vi "Узел обратной связи.vi"() -> ()   [LabVIEW 2017]
doc: "This VI is an exercise in the LabVIEW Basics I course.\n\nIt is used to demonstrate the use of shift registers and feedback nodes. This VI initiallizes a Feedback Node with 1 then multiplies the feedback by 2. Open the block diagram to understand the two methods used."
panel:
  out "Feedback до":dbl
  out "Feedback после":dbl
  # "Этот ВП демонстрирует два способа использования узла обратной связи (Feedback Node). \n \nВ первом случае узел обратной связи отрабатывается после элемента отображения значений функции.\n\nВо втором случае узел обратной связи отрабатывается до элемента отображения значений функции."
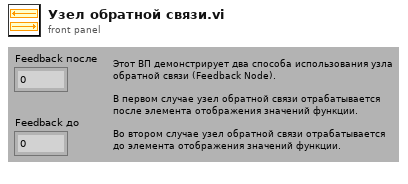
[diagram p1: front panel]
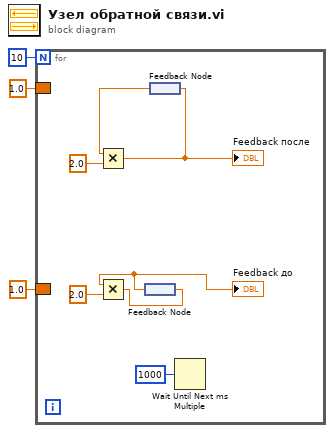
[diagram p0: block diagram]
diagram:
  n1 = for {
    N: 10 -> [_]
    border: 1.0 -> [_]
    border: 1.0 -> [_]
    n2 = feedback #1() -> (w5:dbl)
    "Feedback до" <- w5
    n3 = Multiply(x=w5, y=2.0) -> (x*y=w7:dbl)
    n4 = feedback-in #1(w7) -> ()
    n5 = feedback #2() -> (w9:dbl)
    n6 = Multiply(x=w9, y=2.0) -> (x*y=w4:dbl)
    "Feedback после" <- w4
    n7 = feedback-in #2(w4) -> ()
    n8 = Wait Until Next ms Multiple(millisecond multiple=u32 1000) -> ()  [unwired: 1 out]
  }
